vi "SubVI - Global.vi"() -> ()   [LabVIEW 2017]
panel:
  in  "Histogram Data":i32[](array[numeric])
  in  "Sensor Data":i32[](array[numeric])
  out "Test Running":bool
  in  "Datalog Interval":dbl
  in  "Test Info":string[](array[string])
  in  "File Path":path
  in  "Drive Communication Error":bool
  in  "Start Acquisition ?":bool
  in  "Test Aborted":bool
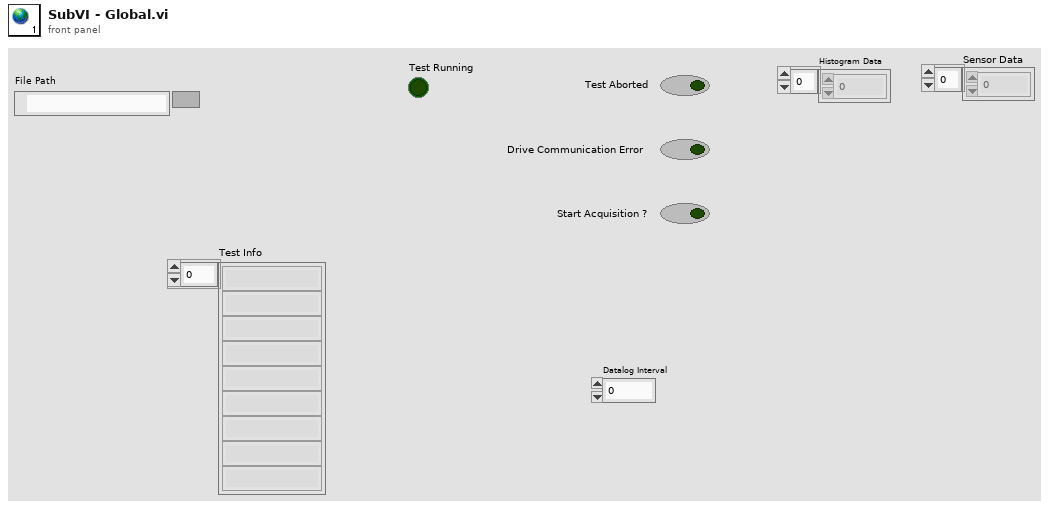
[diagram p1: front panel]
diagram:
